vi "ApplyLayoutToObject.vi"(5 "scaling settings":T1={"scaling factor"={"horizontal"=1.0, "vertical"=1.0}, "scale text"=FALSE} {"scaling factor"."vertical" min=0.0; "scaling factor"."horizontal" min=0.0}, 7 "properties to ignore":variant, 8 "error in (no error)":errorcluster, 10 "GObj Refnum":refnum<vi>, 11 "Boolean Control Layout in":refnum<class "Boolean Control Layout.lvclass">) -> (0 "error out":errorcluster, 3 "Boolean Control Layout out":refnum<class "Boolean Control Layout.lvclass">)   [LabVIEW 2010, in "NI_SE_Front Panel Layout.lvlib" / "Boolean Control Layout.lvclass"]
doc: "Apply layout information to the GObj Refnum."
uses:
  Boolean Control Layout.lvclass
  Scaling Factor_Options.ctl
  XY Scaling Factor.ctl
  Control Layout/Control Layout.lvclass
  Boolean Control Layout.lvclass/Boolean Control Layout.ctl
  Object Layout/Object Layout.lvclass/Object Layout.ctl
  Properties To Ignore.vi
  Set FP Object Size.vi
  NI_SE_Front Panel Layout.lvlib
  Object Layout/Object Layout.lvclass
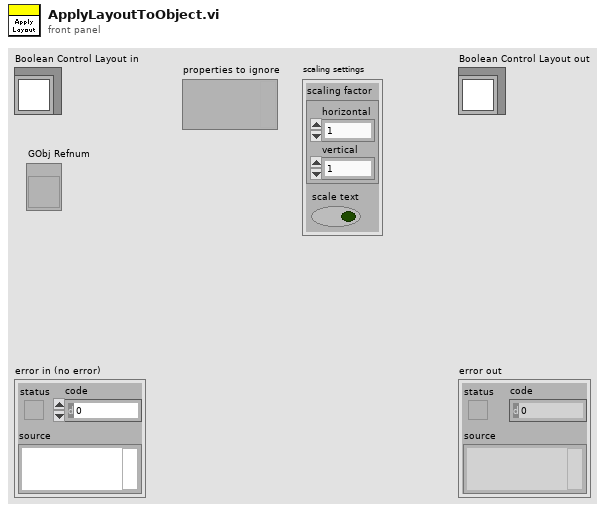
[diagram p1: front panel]
types:
  T1 = typedef "NI_SE_Front Panel Layout.lvlib/Scaling Factor_Options.ctl" = cluster{"scaling factor":T2, "scale text":bool}
  T2 = typedef "NI_SE_Front Panel Layout.lvlib/XY Scaling Factor.ctl" = cluster{"horizontal":dbl, "vertical":dbl}
  T3 = typedef "LVPositionTypeDef.ctl" = cluster{"Left":i32, "Top":i32}
  T4 = typedef "LVBoundsTypeDef.ctl" = cluster{"Width":u32, "Height":u32}
  T5 = typedef "LVRectTypeDef.ctl" = cluster{"Left":i16, "Top":i16, "Right":i16, "Bottom":i16}
  T6 = typedef "LVPointTypeDef.ctl" = cluster{"Horizontal":i16, "Vertical":i16}
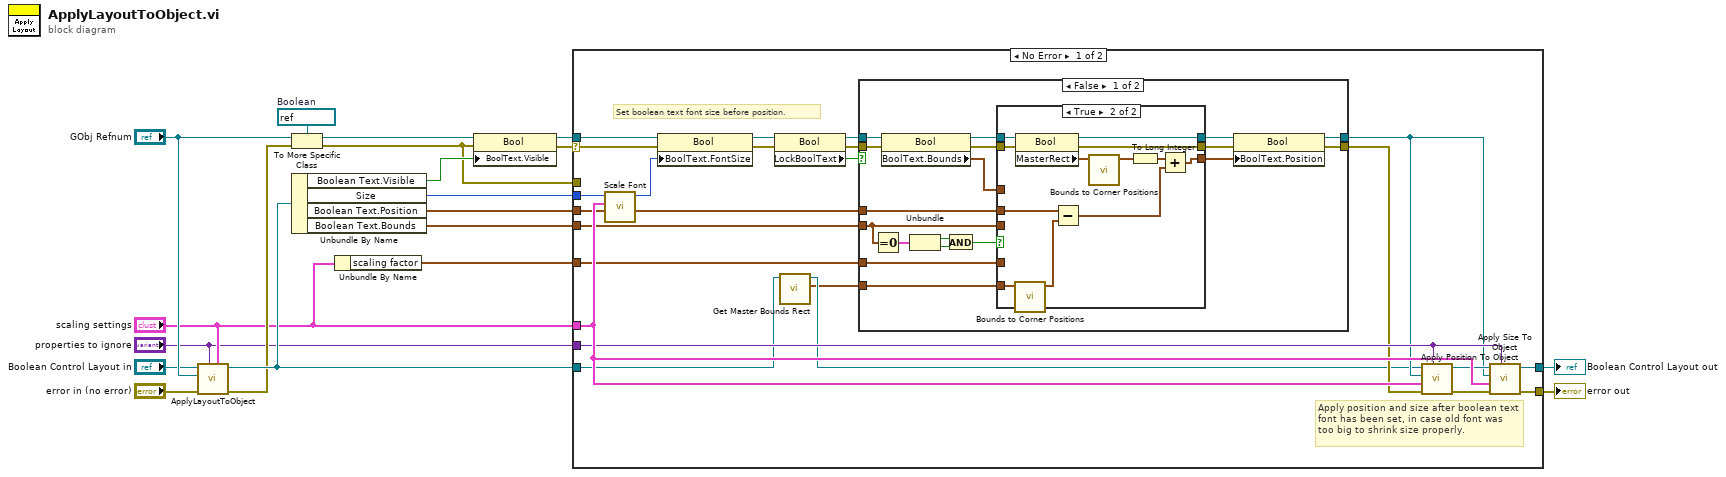
[diagram p0: block diagram]
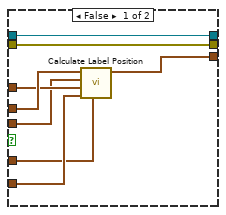
[diagram p2: hidden frame]
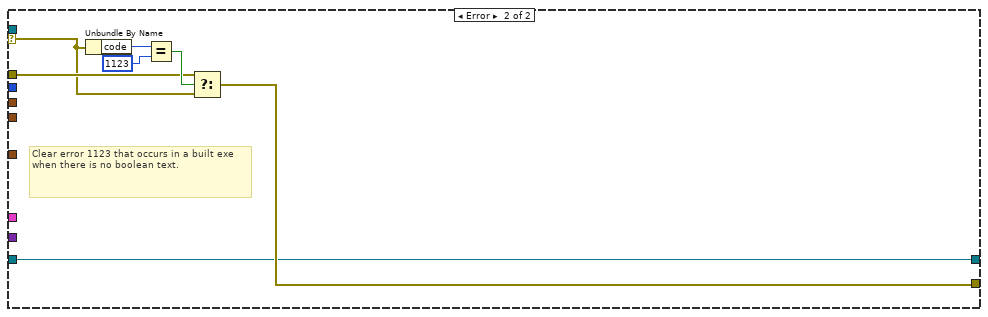
[diagram p4: hidden frame]
diagram:
  w10 = refnum<vi> refnum  # Boolean
  n1 = call-parent "ApplyLayoutToObject.vi"("scaling settings"="scaling settings", "properties to ignore"="properties to ignore", "error in (no error)"="error in (no error)", "GObj Refnum"="GObj Refnum", "Control Layout in"="Boolean Control Layout in") -> ("error out"=w15:errorcluster, "Control Layout out"=w16:refnum<class "Boolean Control Layout.lvclass">)  [unwired: 5 in]
  n2 = To More Specific Class(target class=w10, reference="GObj Refnum", error in=w15) -> (specific class reference=w9:refnum<vi>, error out=w2:errorcluster)
  n3 = Unbundle By Name(w16) -> ("Boolean Text.Visible"=w6:bool, "Size"=w7:u16, "Boolean Text.Position"=w8:T3, "Boolean Text.Bounds"=w1:T4)
  n4 = Unbundle By Name("scaling settings") -> ("scaling factor"=w5:T2)
  n5 = property class="Bool"(reference=w9, error in=w2, "BoolText.Visible"=w6) -> (reference out=w4:refnum<vi>, error out=w3:errorcluster)
  n6 = case shown="No Error" w3 {
    selector: w3 -> [w24 w85]
    tunnel: w16 -> [w22 w83]
    tunnel: [w42 w83] -> w14
    tunnel: [w41 w84] -> w13
    tunnel: "scaling settings" -> [w40 _]
    tunnel: "properties to ignore" -> [w39 _]
    tunnel: w8 -> [w38 _]
    tunnel: w7 -> [w37 _]
    tunnel: w5 -> [w36 _]
    tunnel: w4 -> [w35 _]
    tunnel: w2 -> [_ w86]
    tunnel: w1 -> [w23 _]
    frame No Error {
      # "Set boolean text font size before position."
      # "Apply position and size after boolean text font has been set, in case old font was too big to shrink size properly."
      n7 = call "Scale Font.vi"("scaling settings"=w40, "font size in"=w37) -> ("font size out"=w30:u16)  [unwired: 9 in]
      n8 = property class="Bool"(reference=w35, error in=w24, "BoolText.FontSize"=w30) -> (reference out=w29:refnum<vi>, error out=w26:errorcluster)
      n9 = property class="Bool"(reference=w29, error in=w26) -> (reference out=w28:refnum<vi>, error out=w27:errorcluster, "LockBoolText"=w25:bool)
      n10 = call "Get Master Bounds Rect.vi"("Object Layout in"=w22) -> ("Rect"=w20:T5, "Object Layout out"=w21:refnum<class "Boolean Control Layout.lvclass">)  [unwired: 8 in, 1 out]
      n11 = case shown="False" w25 {
        tunnel: w38 -> [w56 _]
        tunnel: w36 -> [w53 _]
        tunnel: [w60 w82] -> w32
        tunnel: [w59 w81] -> w31
        tunnel: w28 -> [w58 w82]
        tunnel: w27 -> [w57 w81]
        tunnel: w23 -> [w48 _]
        tunnel: w20 -> [w54 _]
        frame False {
          n12 = Equal To 0?(x=w48) -> (x = 0?=w49:cluster{"Width":bool, "Height":bool})
          n13 = property class="Bool"(reference=w58, error in=w57) -> (reference out=w46:refnum<vi>, error out=w44:errorcluster, "BoolText.Bounds"=w55:T4)
          n14 = Unbundle(w49) -> ("Width"=w50:bool, "Height"=w51:bool)
          n15 = And(x=w50, y=w51) -> (x .and. y?=w47:bool)
          n16 = case shown="True" w47 {
            tunnel: w56 -> [w68 w79]
            tunnel: w55 -> [w67 _]
            tunnel: w54 -> [w66 w80]
            tunnel: w53 -> [w65 _]
            tunnel: [w64 w69] -> w52
            tunnel: w48 -> [w63 _]
            tunnel: w46 -> [w62 w77]
            tunnel: [w62 w72] -> w45
            tunnel: w44 -> [w61 w76]
            tunnel: [w61 w73] -> w43
            frame False {
              n17 = call "Calculate Label Position.vi"("scaling factor"=w65, "layout owner bounds"=w66, "scaled object size"=w67, "layout object size"=w63, "layout label position"=w68) -> ("scaled label position"=w64:T3)  [unwired: 6 in]
            }
            frame True {
              n18 = call "Bounds to Corner Positions.vi"("bounds"=w80) -> ("top left"=w78:T6)  [unwired: 9 in, 1 out]
              n19 = property class="Bool"(reference=w77, error in=w76) -> (reference out=w72:refnum<vi>, error out=w73:errorcluster, "MasterRect"=w74:T5)
              n20 = Subtract(x=w79, y=w78) -> (x-y=w70:T3)
              n21 = call "Bounds to Corner Positions.vi"("bounds"=w74) -> ("top left"=w75:T6)  [unwired: 9 in, 1 out]
              n22 = To Long Integer(number=w75) -> (32bit integer=w71:cluster{"Horizontal":i32, "Vertical":i32})
              n23 = Add(x=w71, y=w70) -> (x+y=w69:T3)
            }
          }
          n24 = property class="Bool"(reference=w45, error in=w43, "BoolText.Position"=w52) -> (reference out=w60:refnum<vi>, error out=w59:errorcluster)
        }
        frame True {
        }
      }
      n25 = call "Apply Position To Object.vi"("properties to ignore"=w39, "error in (no error)"=w31, "scaling settings"=w40, "GObj Refnum"=w32, "NI_SE_Object Layout in"=w21) -> ("error out"=w33:errorcluster, "NI_SE_Object Layout out"=w34:refnum<class "Boolean Control Layout.lvclass">)  [unwired: 5 in]
      n26 = call "Apply Size To Object.vi"("properties to ignore"=w39, "error in (no error)"=w33, "scaling settings"=w40, "GObj Refnum"=w32, "NI_SE_Object Layout in"=w34) -> ("error out"=w41:errorcluster, "NI_SE_Object Layout out"=w42:refnum<class "Boolean Control Layout.lvclass">)  [unwired: 5 in]
    }
    frame Error {
      # "Clear error 1123 that occurs in a built exe when there is no boolean text."
      n27 = Unbundle By Name(w85) -> ("code"=w89:i32)
      n28 = Equal?(x=w89, y=1123) -> (x = y?=w87:bool)
      n29 = Select(t=w86, s=w87, f=w85) -> (s? t:f=w84:errorcluster)
    }
  }
  "error out" <- w13
  "Boolean Control Layout out" <- w14
